vi "Range_to_memory_address_CH0.vi"(11 "Range IN1":dbl) -> (0 "LB address":string, 1 "HB address":string, 2 "UB address":string, 3 "MB address":string, 4 "Sign Addrss":string)   [LabVIEW 2012]
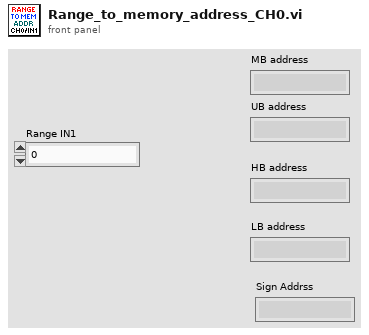
[diagram p1: front panel]
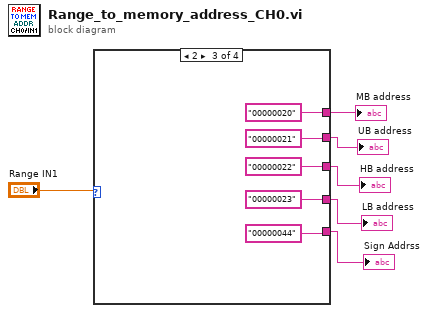
[diagram p0: block diagram]
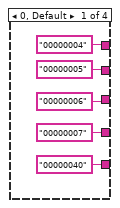
[diagram p2: hidden frame]
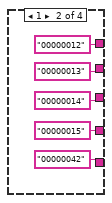
[diagram p3: hidden frame]
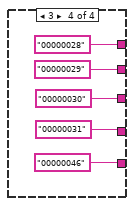
[diagram p4: hidden frame]
diagram:
  n1 = case shown="2" "Range IN1" {
    tunnel: ["00000004" "00000012" "00000020" "00000028"] -> w5
    tunnel: ["00000005" "00000013" "00000021" "00000029"] -> w4
    tunnel: ["00000006" "00000014" "00000022" "00000030"] -> w3
    tunnel: ["00000007" "00000015" "00000023" "00000031"] -> w2
    tunnel: ["00000040" "00000042" "00000044" "00000046"] -> w1
    frame 0, Default {
    }
    frame 1 {
    }
    frame 2 {
    }
    frame 3 {
    }
  }
  "MB address" <- w5
  "UB address" <- w4
  "HB address" <- w3
  "LB address" <- w2
  "Sign Addrss" <- w1
